vi "Export_Positions.vi"(0 "Boolean":bool) -> ()   [LabVIEW 2013]
uses:
  <vilib>/Utility/file.llb/Write To Spreadsheet File (DBL).vi
panel:
  in  "File Path":path
  out "P10":dbl[](array[numeric])
  out "P9":dbl[](array[numeric])
  out "P8":dbl[](array[numeric])
  out "P6":dbl[](array[numeric])
  out "P5":dbl[](array[numeric])
  out "P4":dbl[](array[numeric])
  out "P7":dbl[](array[numeric])
  out "P3":dbl[](array[numeric])
  out "P2":dbl[](array[numeric])
  out "P1":dbl[](array[numeric])
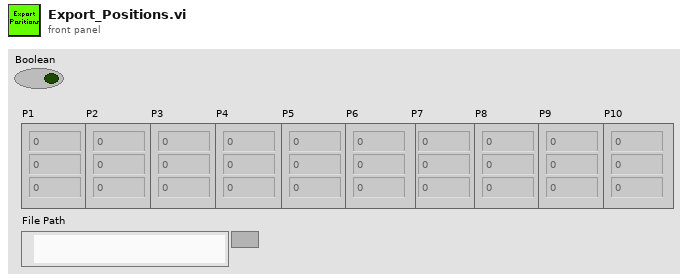
[diagram p1: front panel]
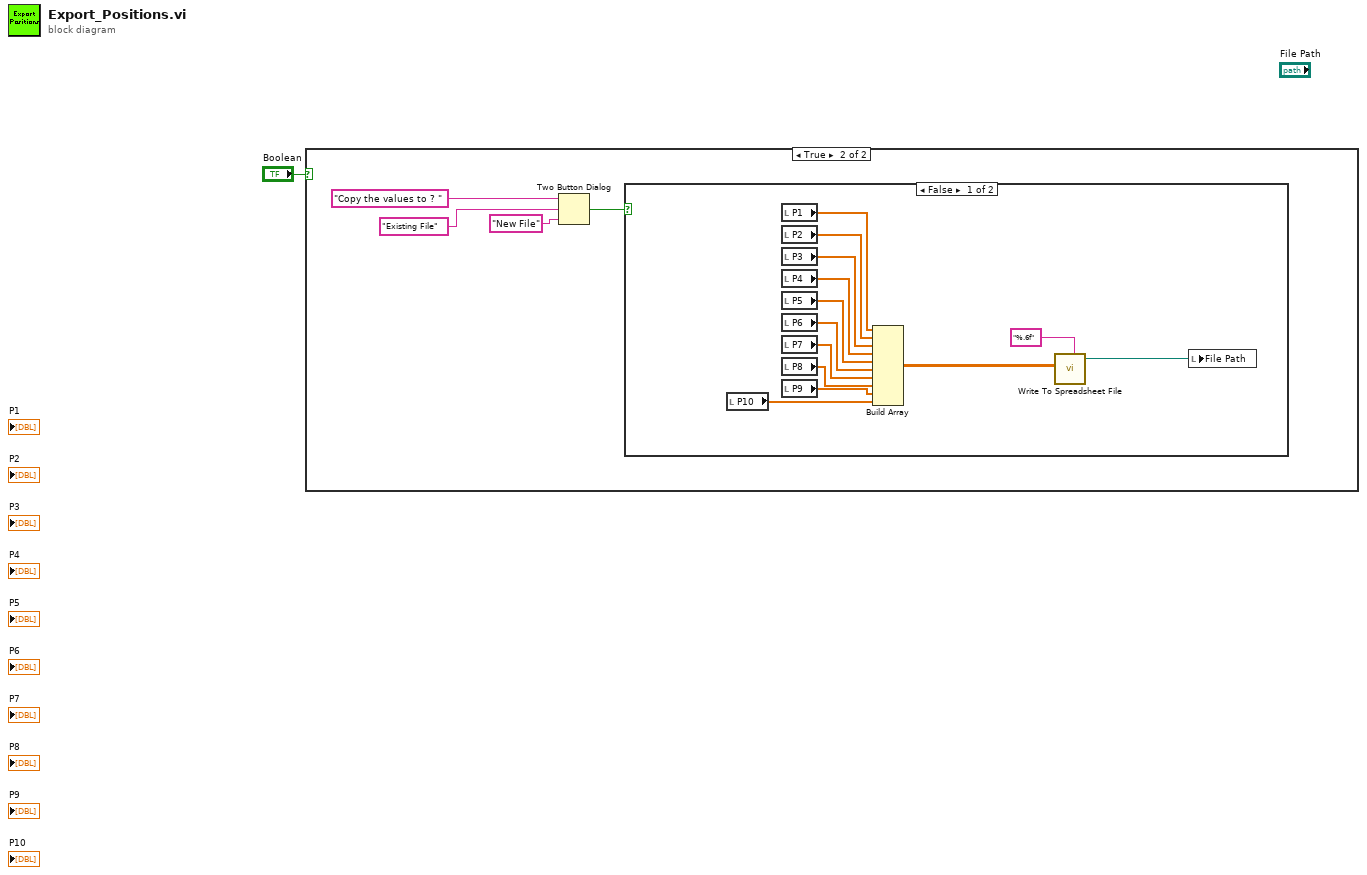
[diagram p0: block diagram]
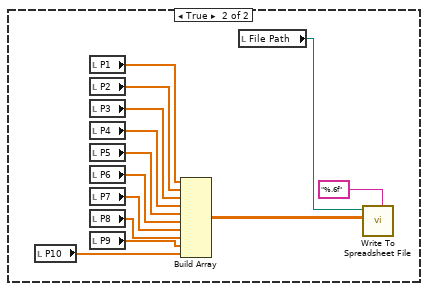
[diagram p3: hidden frame]
diagram:
  n1 = case shown="True" "Boolean" {
    frame False {
    }
    frame True {
      n2 = Two Button Dialog(message="Copy the values to ? ", 1:"New File" ("F button name (\"Cancel\")"), 2:"Existing File" ("T button name (\"OK\")")) -> (T button?=w2:bool)
      n3 = case shown="False" w2 {
        frame False {
          n4 = local read "P10"() -> (w12:dbl[])
          n5 = local read "P1"() -> (w18:dbl[])
          n6 = local read "P2"() -> (w17:dbl[])
          n7 = local read "P3"() -> (w16:dbl[])
          n8 = local read "P4"() -> (w15:dbl[])
          n9 = local read "P5"() -> (w14:dbl[])
          n10 = local read "P6"() -> (w13:dbl[])
          n11 = local read "P7"() -> (w9:dbl[])
          n12 = local read "P8"() -> (w10:dbl[])
          n13 = local read "P9"() -> (w11:dbl[])
          n14 = Build Array(w18, w17, w16, w15, w14, w13, w9, w10, w11, w12) -> (w6:dbl[][])
          n15 = call-poly <vilib>:"Write To Spreadsheet File.vi"("format (%.3f)"="%.6f", "2D data"=w6) -> ("new file path (Not A Path if cancelled)"=w8:path)  [unwired: 6 in]
          n16 = local write "File Path"(w8) -> ()
        }
        frame True {
          n17 = local read "P10"() -> (w20:dbl[])
          n18 = local read "P1"() -> (w21:dbl[])
          n19 = local read "P2"() -> (w22:dbl[])
          n20 = local read "P3"() -> (w23:dbl[])
          n21 = local read "P4"() -> (w24:dbl[])
          n22 = local read "P5"() -> (w25:dbl[])
          n23 = local read "P6"() -> (w26:dbl[])
          n24 = local read "P7"() -> (w27:dbl[])
          n25 = local read "P8"() -> (w28:dbl[])
          n26 = local read "P9"() -> (w29:dbl[])
          n27 = Build Array(w21, w22, w23, w24, w25, w26, w27, w28, w29, w20) -> (w30:dbl[][])
          n28 = local read "File Path"() -> (w19:path)
          n29 = call-poly <vilib>:"Write To Spreadsheet File.vi"("format (%.3f)"="%.6f", "2D data"=w30, "file path (dialog if empty)"=w19) -> ()  [unwired: 5 in, 1 out]
        }
      }
    }
  }
